vi "emi_Drive Path from driver Letter.vi"(7 "Drive letter":string) -> (8 "Path":path)   [LabVIEW 2010]
doc: "convert a string containing the drive letter, to teh root path of the driver.\n\nC-> C:/"
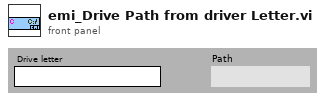
[diagram p1: front panel]
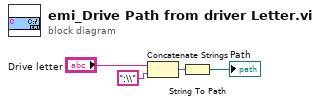
[diagram p0: block diagram]
diagram:
  n1 = Concatenate Strings("Drive letter", ":\\" ("string")) -> (w2:string)
  n2 = String To Path(string=w2) -> (path=→"Path":path)
